vi "Write Gas Ref.vi"(8 "error in (no error)":errorcluster, 10 "Gas Ref":refnum<data-value>, 11 "DMA in":refnum<class "DMA.lvclass">) -> (0 "error out":errorcluster, 3 "DMA out":refnum<class "DMA.lvclass">)   [LabVIEW 2014, in "DMA.lvclass"]
uses:
  DMA.lvclass
  Atmospheric/Gas Properties/Gas Properties.lvclass
  DMA.lvclass/DMA.ctl
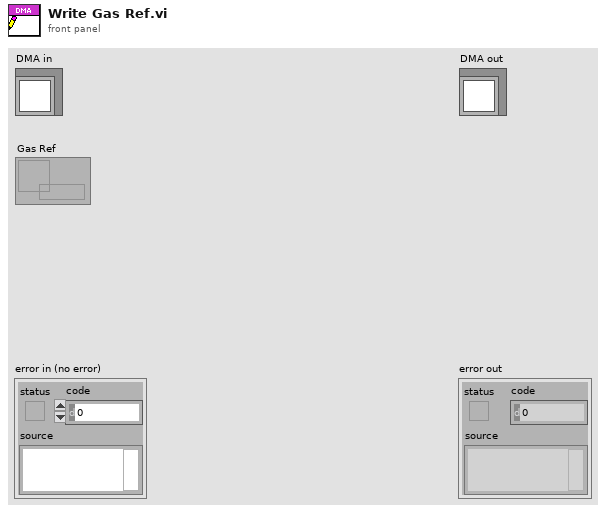
[diagram p1: front panel]
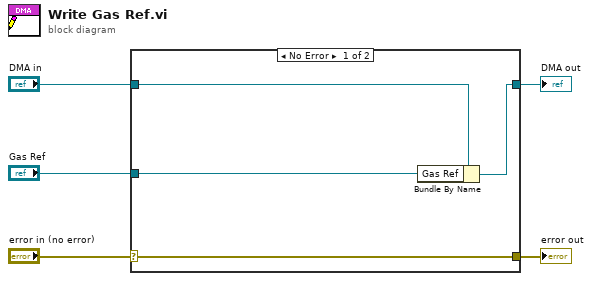
[diagram p0: block diagram]
diagram:
  n1 = case shown="No Error" "error in (no error)" {
    selector: "error in (no error)" -> [w9 w10]
    tunnel: [w9 w10] -> w4
    tunnel: [w7 w11] -> w2
    tunnel: "DMA in" -> [w8 w11]
    tunnel: "Gas Ref" -> [w6 _]
    frame No Error {
      n2 = Bundle By Name(cluster=w8, "Gas Ref"=w6) -> (w7:refnum<class "DMA.lvclass">)
    }
    frame Error {
    }
  }
  "error out" <- w4
  "DMA out" <- w2
